vi "gentec-SOLO_PE.Basic Read.vi"(8 "error in (no error)":errorcluster, 10 "byte count":u32, 11 "VISA Refnum in":refnum<visa-resource-name>) -> (0 "error out":errorcluster, 1 "Timeout?":bool, 2 "read buffer":string, 3 "VISA Refnum out":refnum<visa-resource-name>)   [LabVIEW 2014, in "gentec-SOLO-PE - Driver.lvlib"]
doc: "This VI calls a VISA Read, adds a delay and handles certain VISA Errors."
uses:
  gentec-SOLO-PE - Driver.lvlib
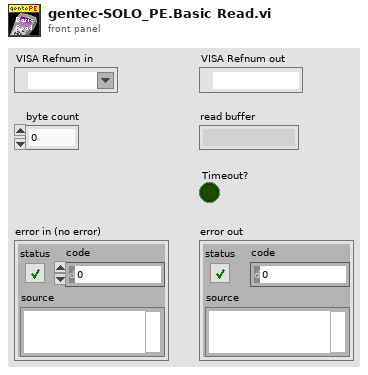
[diagram p1: front panel]
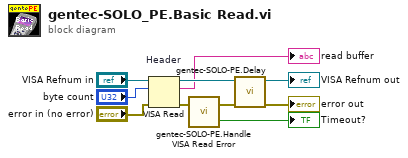
[diagram p0: block diagram]
diagram:
  n1 = VISA Read "Header"(VISA resource name="VISA Refnum in", byte count="byte count", error in (no error)="error in (no error)") -> (VISA resource name out=w7:refnum<visa-resource-name>, read buffer=→"read buffer":string, error out=w6:errorcluster)  [unwired: 1 out]
  n2 = call "gentec-SOLO-PE.Handle VISA Read Error.vi"("error in"=w6) -> ("Timeout?"=→"Timeout?":bool, "error out"=w9:errorcluster)  [unwired: 1 in]
  n3 = call "gentec-SOLO-PE.Delay.vi"("error in (no error)"=w9, "VISA resource In"=w7) -> ("error out"=→"error out":errorcluster, "VISA resource Out"=→"VISA Refnum out":refnum<visa-resource-name>)  [unwired: 4 in]
